vi "Continous Message Test.vi"(6 "timeout(s)":dbl=5.0, 11 "Sequence Context In":refnum<k7>) -> ()   [LabVIEW 2020]
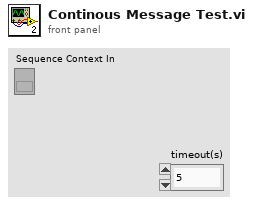
[diagram p1: front panel]
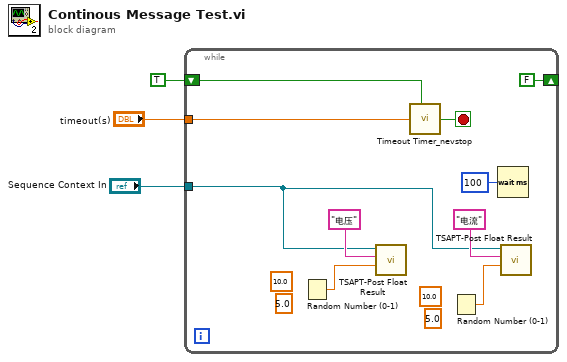
[diagram p0: block diagram]
diagram:
  n1 = while {
    tunnel: "timeout(s)" -> [w13]
    shift-right: [FALSE ("reset?(F)")] -> _
    shift-left: TRUE ("reset?(F)") -> [w12]
    tunnel: "Sequence Context In" -> [w4]
    stop <- w11 stop-if-true
    (unwired) 5.0 ("Low")
    (unwired) 10.0 ("High")
    (unwired) 5.0 ("Low")
    (unwired) 10.0 ("High")
    n2 = Random Number (0-1)() -> (number: 0 to 1=w7:dbl)
    n3 = call "TSAPT-Post Float Result.vi"("Result"=w7, "Name"="电压", "Sequence Context In"=w4) -> ()  [unwired: 8 in, 1 out]
    n4 = call <userlib>:"Timeout Timer_nevstop.vi"("reset?(F)"=w12, "timeout(s)"=w13) -> ("timeout?"=w11:bool)  [unwired: 6 in, 1 out]
    n5 = Random Number (0-1)() -> (number: 0 to 1=w6:dbl)
    n6 = Wait (ms)(milliseconds to wait=u32 100) -> ()  [unwired: 1 out]
    n7 = call "TSAPT-Post Float Result.vi"("Result"=w6, "Name"="电流", "Sequence Context In"=w4) -> ()  [unwired: 8 in, 1 out]
  }
